vi "svx_Create Indic (Rev).vi"(5 "reset?(F)":bool, 8 "error in (no error)":errorcluster, 9 "segment settings":cluster{"start [rev]":dbl, "end [rev]":dbl}, 10 "actual samples/rev":dbl format="%.2f", 11 "interpolated pulse positions in":dbl[](array[numeric])) -> (0 "error out":errorcluster, 1 "indice":cluster{"start":i32, "length":i32}, 2 "actual samples/rev out":dbl format="%.2f", 3 "interpolated pulse positions out":dbl[](array[numeric]), 4 "end reached":bool)   [LabVIEW 2017]
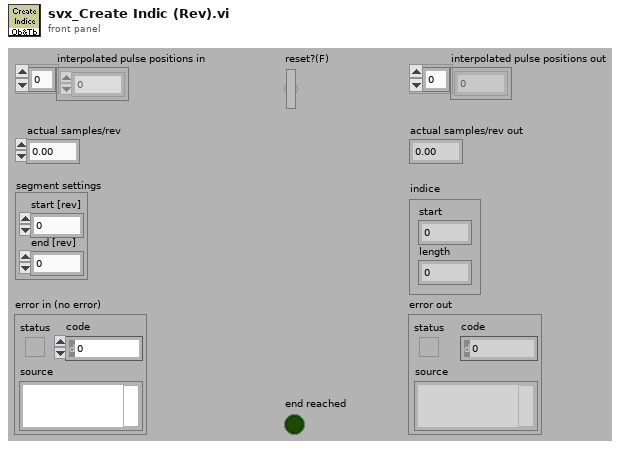
[diagram p1: front panel]
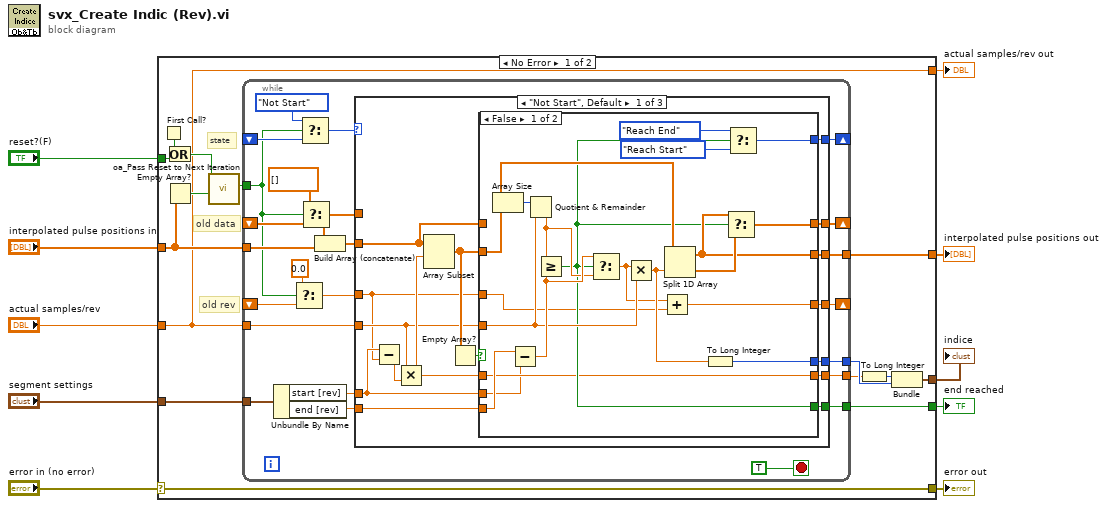
[diagram p0: block diagram]
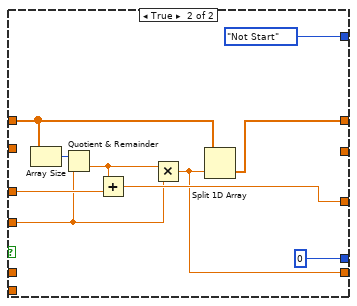
[diagram p2: hidden frame]
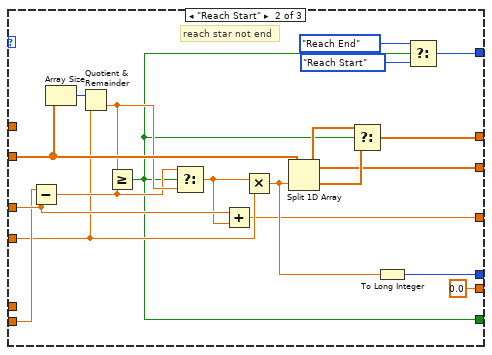
[diagram p3: hidden frame]
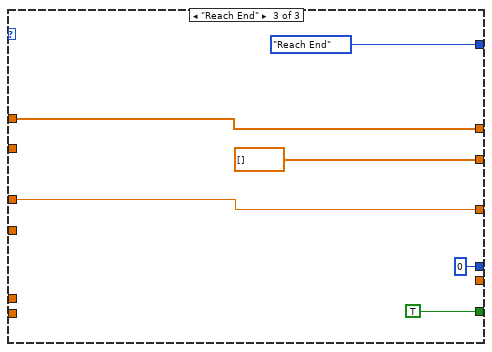
[diagram p4: hidden frame]
diagram:
  n1 = case shown="No Error" "error in (no error)" {
    selector: "error in (no error)" -> [w25 w121]
    tunnel: [w25 w121] -> w9
    tunnel: "reset?(F)" -> [w24 _]
    tunnel: "interpolated pulse positions in" -> [w17 _]
    tunnel: "segment settings" -> [w21 _]
    tunnel: "actual samples/rev" -> [w15 _]
    tunnel: [w19 _] -> w4
    tunnel: [w18 _] -> w3
    tunnel: [w15 _] -> w2
    tunnel: [w11 _] -> w1
    frame No Error {
      # "old rev"
      # "old data"
      # "state"
      n2 = First Call?() -> (First Call?: T/F=w23:bool)
      n3 = Or(x=w23, y=w24) -> (x .or. y?=w22:bool)
      n4 = Empty Array?(array=w17) -> (empty?=w16:bool)
      n5 = call <vilib>:"oa_Pass Reset to Next Iteration.vi"("trigger"=w16, "reset?(F)"=w22) -> ("reset out"=w20:bool)  [unwired: 9 in]
      n6 = while {
        shift-right: [w37] -> _
        shift-left: _ -> [w32]
        tunnel: w21 -> [w48]
        tunnel: w20 -> [w31]
        tunnel: w17 -> [w45]
        tunnel: w15 -> [w47]
        shift-right: [w36] -> _
        shift-left: _ -> [w46]
        shift-right: [w38] -> _
        shift-left: _ -> [w42]
        tunnel: [w35] -> w19
        tunnel: [w27] -> w18
        tunnel: [w28] -> w14
        tunnel: [w26] -> w13
        stop <- TRUE stop-if-true
        n7 = Unbundle By Name(w48) -> ("start [rev]"=w33:dbl, "end [rev]"=w40:dbl)
        n8 = Select(t=0.0 ("end [rev]"), s=w31, f=w42) -> (s? t:f=w39:dbl)
        n9 = Select(t=enum16{"Not Start", "Reach Start", "Reach End"}."Not Start" ("Enum"), s=w31, f=w32) -> (s? t:f=w29:enum16{"Not Start", "Reach Start", "Reach End"})
        n10 = Select(t=dbl[] [] ("interpolated pulse positions out"), s=w31, f=w46) -> (s? t:f=w34:dbl[])
        n11 = Build Array (concatenate)(w34, w45) -> (w44:dbl[])
        n12 = case shown="\"Not Start\", Default" w29 {
          tunnel: w44 -> [w63 w114 _]
          tunnel: w47 -> [w53 w101 _]
          tunnel: w40 -> [w59 w112 _]
          tunnel: w39 -> [w51 w113 w118]
          tunnel: [w60 w96 w118] -> w38
          tunnel: [w64 w104 enum16{"Not Start", "Reach Start", "Reach End"}."Reach End" ("Enum")] -> w37
          tunnel: [w62 w103 w120] -> w36
          tunnel: [w61 w102 dbl[] [] ("interpolated pulse positions out")] -> w35
          tunnel: w34 -> [_ _ w120]
          tunnel: w33 -> [w52 _ _]
          tunnel: [w57 w100 TRUE ("end reach?")] -> w27
          tunnel: [w56 w98 0] -> w28
          tunnel: [w54 0.0 _] -> w26
          frame "Not Start", Default {
            n13 = Subtract(x=w52, y=w51) -> (x-y=w50:dbl)
            n14 = Multiply(x=w53, y=w50) -> (x*y=w55:dbl)
            n15 = Array Subset(array=w63, index=w55) -> (w58:dbl[])  [unwired: 1 in]
            n16 = Empty Array?(array=w58) -> (empty?=w65:bool)
            n17 = case shown="False" w65 {
              tunnel: [w75 enum16{"Not Start", "Reach Start", "Reach End"}."Not Start" ("Enum")] -> w64
              tunnel: [w78 w87] -> w62
              tunnel: w63 -> [_ w88]
              tunnel: [w79 _] -> w61
              tunnel: [w67 w91] -> w60
              tunnel: w59 -> [w84 _]
              tunnel: w51 -> [w68 w92]
              tunnel: w58 -> [w81 _]
              tunnel: w53 -> [w77 w89]
              tunnel: w52 -> [w66 _]
              tunnel: [w72 _] -> w57
              tunnel: [w71 0] -> w56
              tunnel: w55 -> [w70 _]
              tunnel: [w70 w86] -> w54
              frame False {
                n18 = Array Size(array=w81) -> (size(s)=w85:i32)
                n19 = Subtract(x=w84, y=w66) -> (x-y=w83:dbl)
                n20 = Quotient & Remainder(x=w85, y=w77) -> (floor(x/y)=w82:dbl)  [unwired: 1 out]
                n21 = Greater Or Equal?(x=w82, y=w83) -> (x >= y?=w72:bool)
                n22 = Select(t=w83, s=w72, f=w82) -> (s? t:f=w69:dbl)
                n23 = Multiply(x=w69, y=w77) -> (x*y=w73:dbl)
                n24 = Add(x=w69, y=w68) -> (x+y=w67:dbl)
                n25 = Split 1D Array(array=w81, index=w73) -> (first subarray=w79:dbl[], second subarray=w80:dbl[])
                n26 = To Long Integer(number=w73) -> (32bit integer=w71:i32)
                n27 = Select(t=w79, s=w72, f=w80) -> (s? t:f=w78:dbl[])
                n28 = Select(t=enum16{"Not Start", "Reach Start", "Reach End"}."Reach End" ("Enum"), s=w72, f=enum16{"Not Start", "Reach Start", "Reach End"}."Reach Start") -> (s? t:f=w75:enum16{"Not Start", "Reach Start", "Reach End"})
              }
              frame True {
                n29 = Array Size(array=w88) -> (size(s)=w93:i32)
                n30 = Quotient & Remainder(x=w93, y=w89) -> (floor(x/y)=w90:dbl)  [unwired: 1 out]
                n31 = Add(x=w90, y=w92) -> (x+y=w91:dbl)
                n32 = Multiply(x=w90, y=w89) -> (x*y=w86:dbl)
                n33 = Split 1D Array(array=w88, index=w86) -> (second subarray=w87:dbl[])  [unwired: 1 out]
              }
            }
          }
          frame "Reach Start" {
            # "reach star not end"
            n34 = Subtract(x=w112, y=w113) -> (x-y=w108:dbl)
            n35 = Array Size(array=w114) -> (size(s)=w111:i32)
            n36 = Quotient & Remainder(x=w111, y=w101) -> (floor(x/y)=w110:dbl)  [unwired: 1 out]
            n37 = Greater Or Equal?(x=w110, y=w108) -> (x >= y?=w100:bool)
            n38 = Select(t=w108, s=w100, f=w110) -> (s? t:f=w109:dbl)
            n39 = Add(x=w113, y=w109) -> (x+y=w96:dbl)
            n40 = Multiply(x=w109, y=w101) -> (x*y=w99:dbl)
            n41 = Split 1D Array(array=w114, index=w99) -> (first subarray=w102:dbl[], second subarray=w107:dbl[])
            n42 = Select(t=w102, s=w100, f=w107) -> (s? t:f=w103:dbl[])
            n43 = To Long Integer(number=w99) -> (32bit integer=w98:i32)
            n44 = Select(t=enum16{"Not Start", "Reach Start", "Reach End"}."Reach End" ("Enum"), s=w100, f=enum16{"Not Start", "Reach Start", "Reach End"}."Reach Start") -> (s? t:f=w104:enum16{"Not Start", "Reach Start", "Reach End"})
          }
          frame "Reach End" {
          }
        }
      }
      n45 = To Long Integer(number=w13) -> (32bit integer=w12:i32)
      n46 = Bundle(w12, w14) -> (w11:cluster{i32, i32})  [unwired: 1 in]
    }
    frame Error {
    }
  }
  "error out" <- w9
  "interpolated pulse positions out" <- w4
  "end reached" <- w3
  "actual samples/rev out" <- w2
  "indice" <- w1
